vi "ATM.vi"() -> ()   [LabVIEW 2015]
uses:
  all data.ctl
  User data.ctl
  status.ctl
  user action.ctl
panel:
  out "error out":errorcluster
  in  "error in":errorcluster
  in  "Enter":bool
  in  "User Input":string
  in  "Right Buttons":T1
  out "Right Menu":T2
  in  "Left Buttons":T1
  out "Left Menu":T2
  in  "Card Simulator":bool
  out "ATM Messages":string
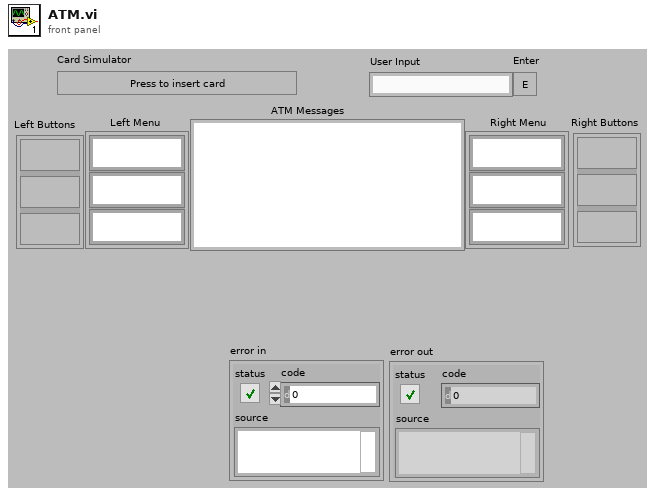
[diagram p1: front panel]
types:
  T1 = cluster{"Func Button":bool, "Func Button 2":bool, "Func Button 3":bool}
  T2 = cluster{"RFS String":string, "RFS String 2":string, "RFS String 3":string}
  T3 = enum8{"Enabled", "Disabled", "Disabled and Grayed Out"}
  T4 = typedef "all data.ctl" = cluster{"order":string, "Users":T5[], "user num":i32}
  T5 = typedef "User data.ctl" = cluster{"Code":string, "Name":string, "Surname":string, "Money":string}
  T6 = typedef "status.ctl" = enum16{"Get", "Set"}
  T7 = typedef "user action.ctl" = enum16{"Name", "Withdraw", "Deposit", "Balance"}
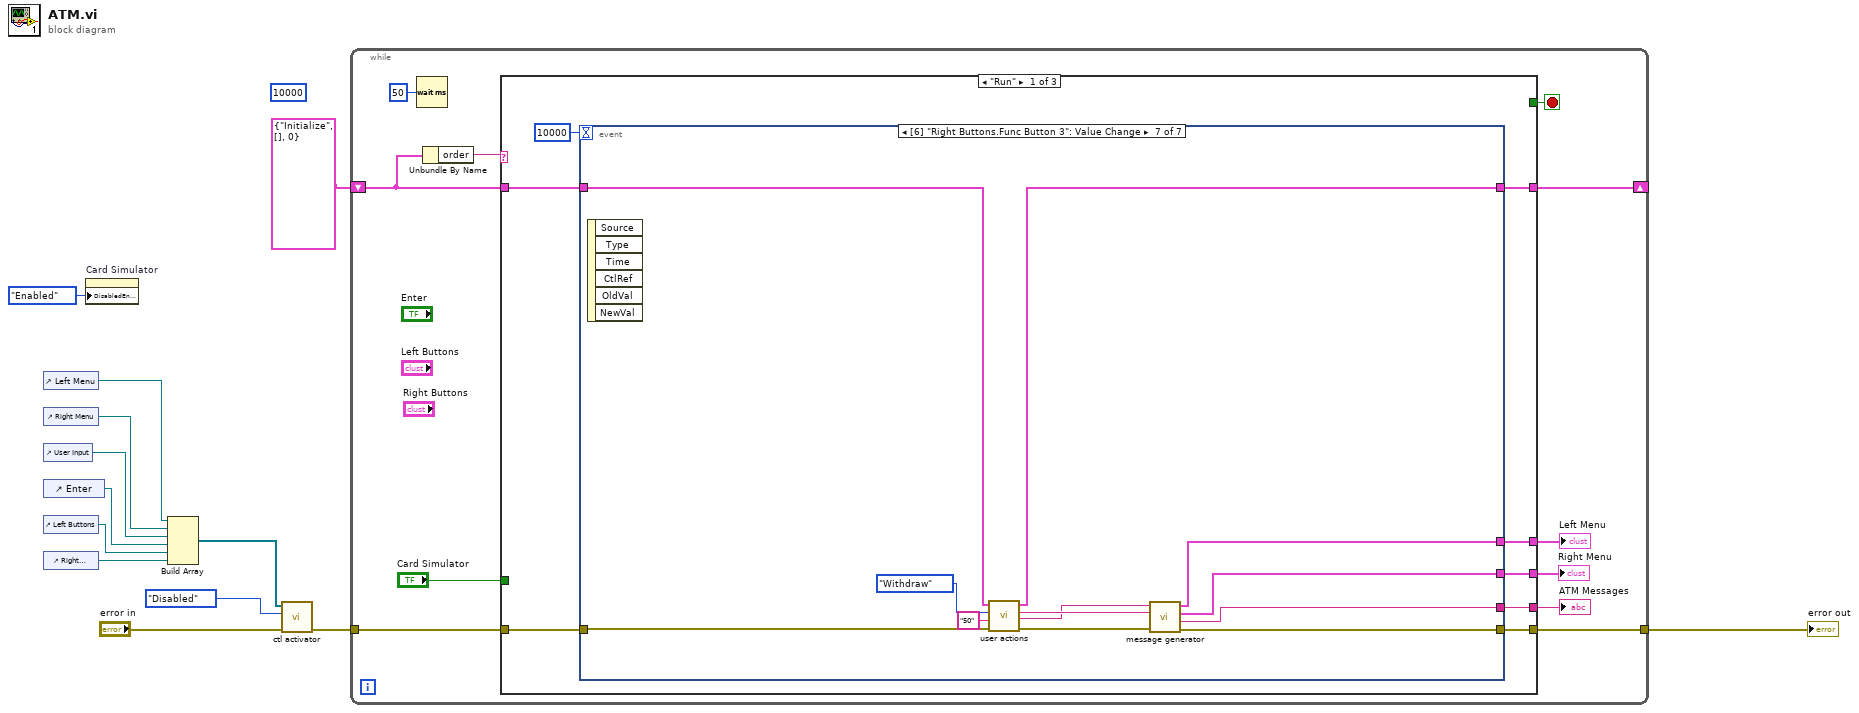
[diagram p0: block diagram]
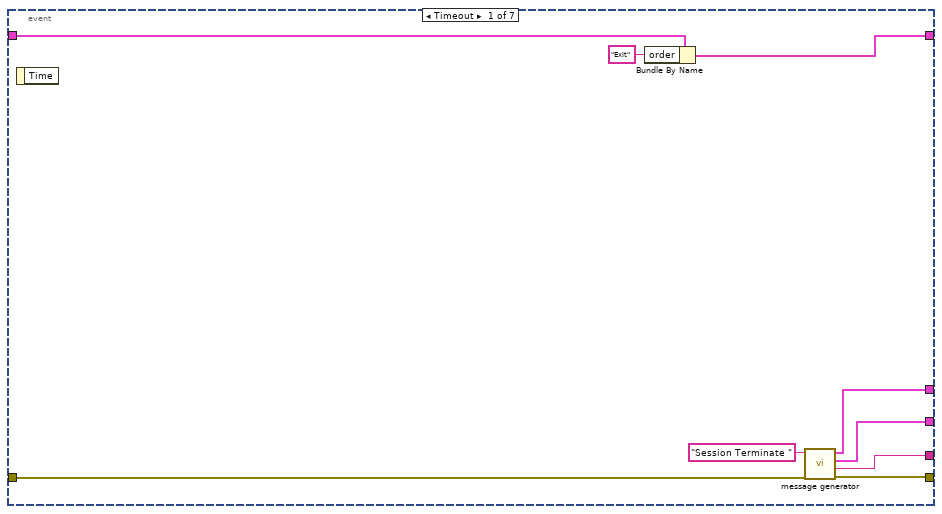
[diagram p2: hidden frame]
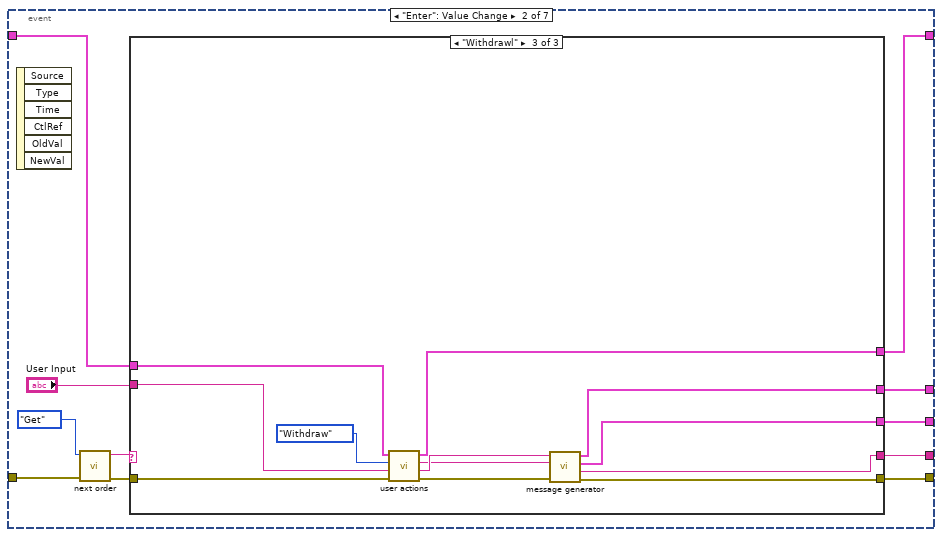
[diagram p3: hidden frame]
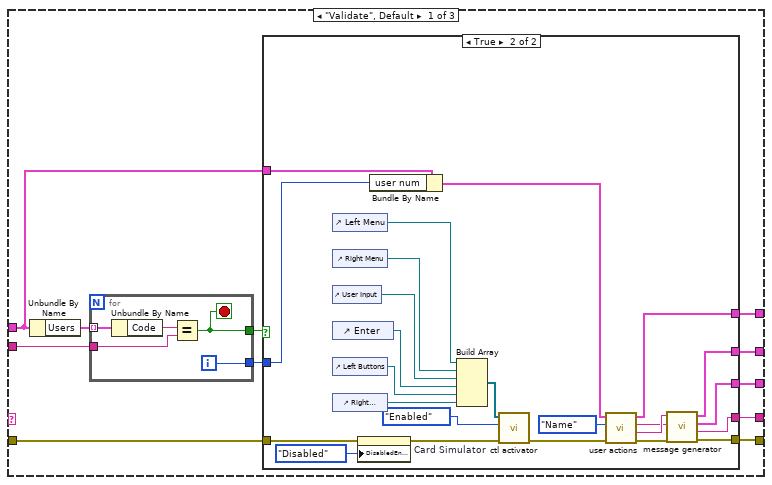
[diagram p4: hidden frame]
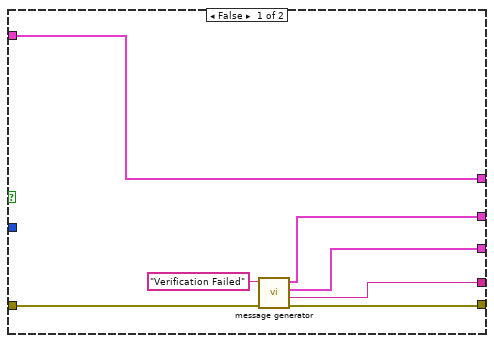
[diagram p5: hidden frame]
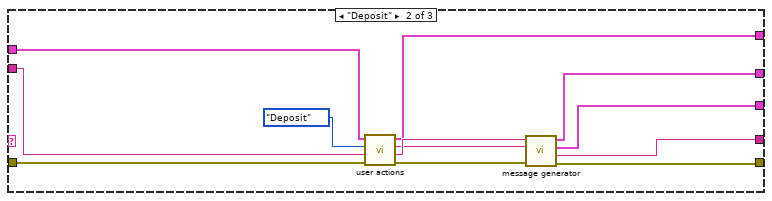
[diagram p6: hidden frame]
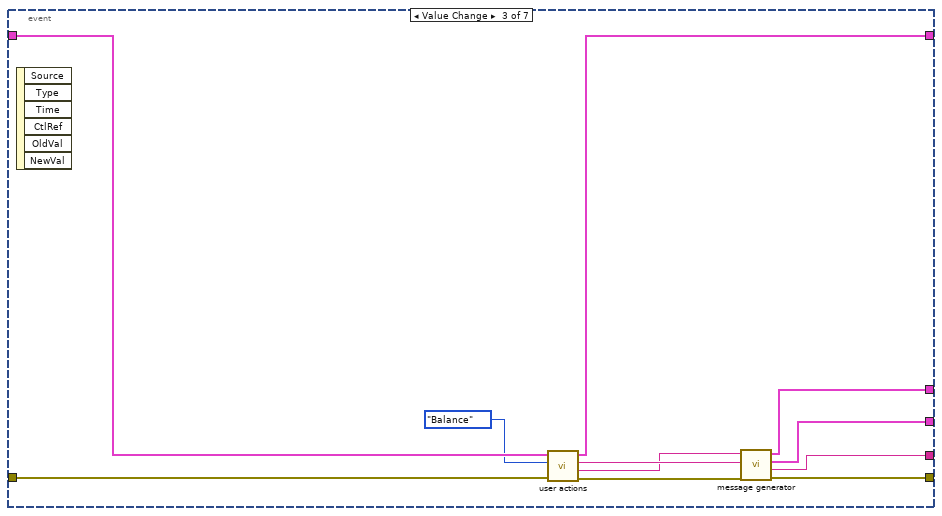
[diagram p7: hidden frame]
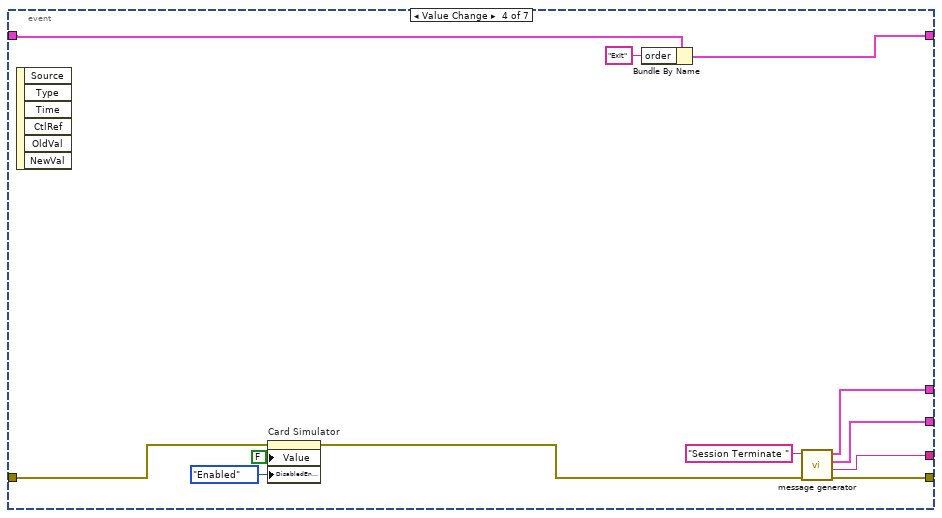
[diagram p8: hidden frame]
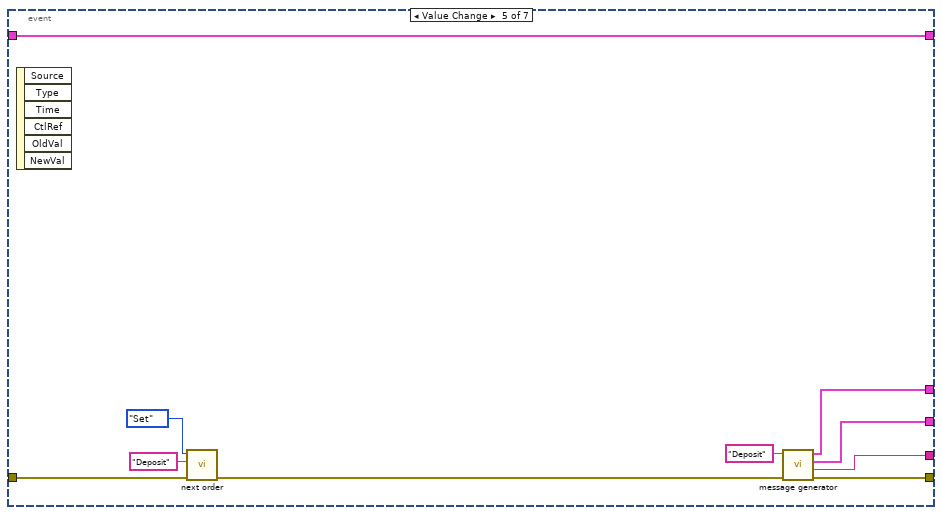
[diagram p9: hidden frame]
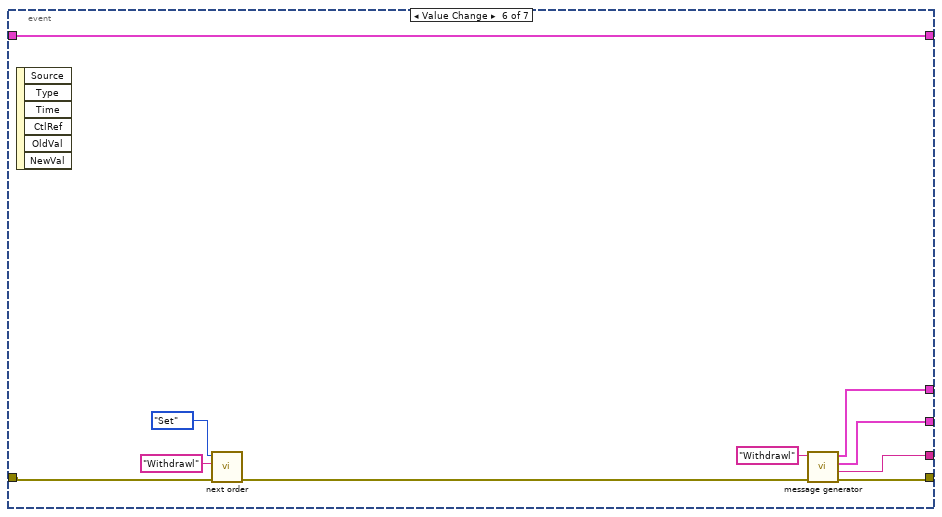
[diagram p10: hidden frame]
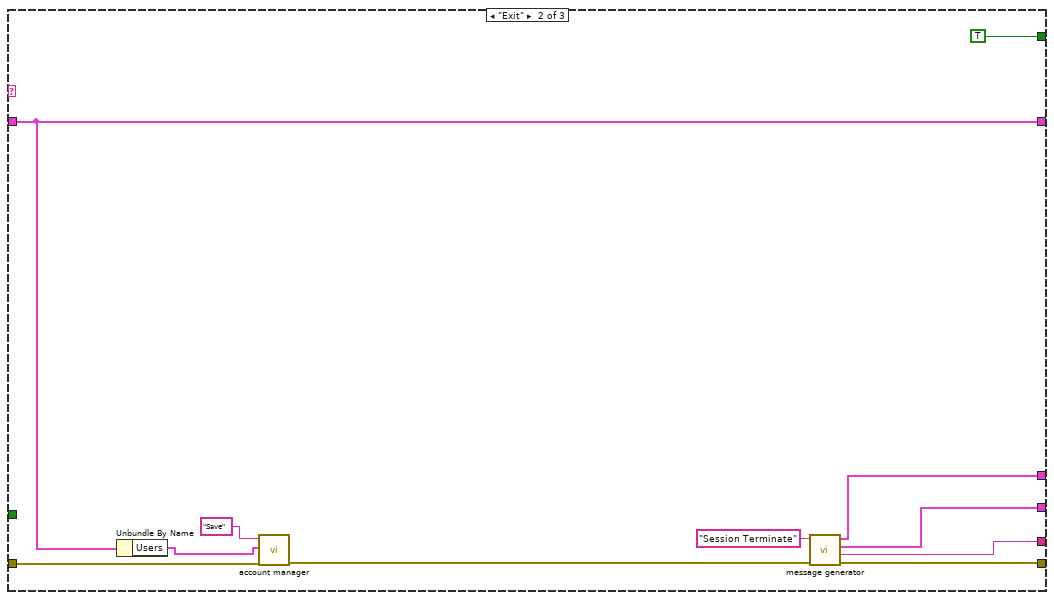
[diagram p11: hidden frame]
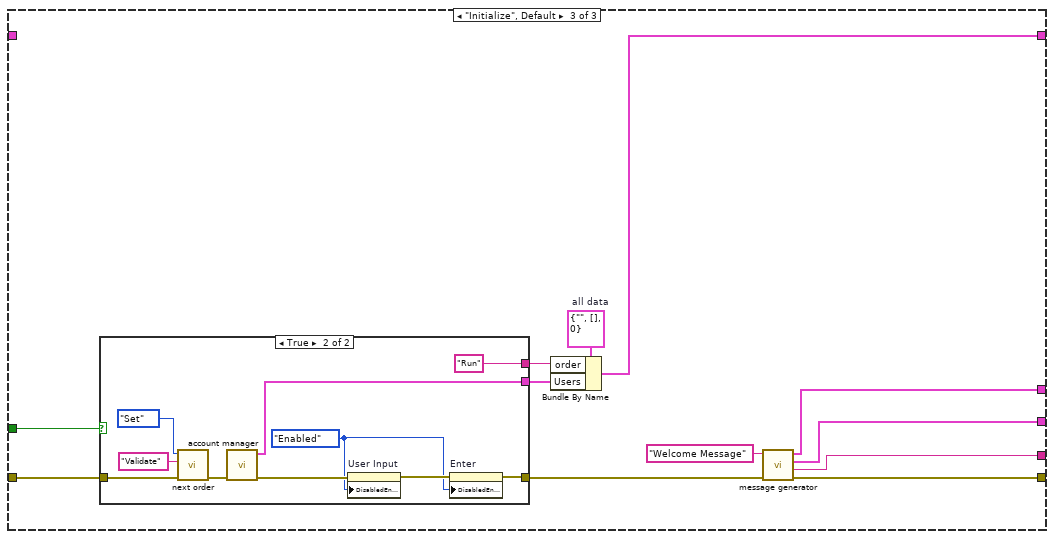
[diagram p12: hidden frame]
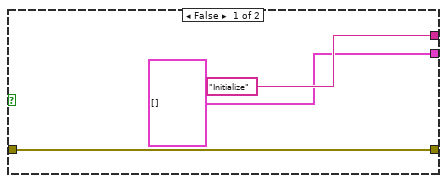
[diagram p13: hidden frame]
diagram:
  (unwired) 10000
  n1 = control-ref of="Left Menu"() -> (w4:refnum<vi>)
  n2 = control-ref of="Right Menu"() -> (w3:refnum<vi>)
  n3 = control-ref of="User Input"() -> (w5:refnum<vi>)
  n4 = control-ref of="Enter"() -> (w6:refnum<vi>)
  n5 = control-ref of="Left Buttons"() -> (w7:refnum<vi>)
  n6 = control-ref of="Right Buttons"() -> (w8:refnum<vi>)
  n7 = property on="Card Simulator" class="Bool (strict)"("DisabledEnum"=T3."Enabled" ("Disabled")) -> ()  [unwired: 2 in, 2 out]
  n8 = Build Array(w4, w3, w5, w6, w7, w8) -> (w2:refnum<vi>[])
  n9 = call "ctl activator.vi"("error in"="error in", "Disabled"=T3."Disabled", "Array"=w2) -> ("error out"=w10:errorcluster)  [unwired: 8 in]
  n10 = while {
    tunnel: w10 -> [w24]
    tunnel: [w21] -> w13
    shift-right: [w23] -> _
    shift-left: T4 {"order"="Initialize", "Users"=[], "user num"=0} ("all data") -> [w15]
    stop <- w16 stop-if-true
    n11 = Wait (ms)(milliseconds to wait=u32 50) -> ()  [unwired: 1 out]
    n12 = Unbundle By Name(w15) -> ("order"=w20:string)
    n13 = case shown="\"Run\"" w20 {
      tunnel: w24 -> [w32 w188 w200]
      tunnel: [w26 w186 w197] -> w23
      tunnel: "Card Simulator" -> [_ _ w196]
      tunnel: [w31 w183 w194] -> w21
      tunnel: [w28 w179 w192] -> w19
      tunnel: [w29 w180 w191] -> w18
      tunnel: [w30 w181 w190] -> w17
      tunnel: [_ TRUE _] -> w16
      tunnel: w15 -> [w27 w186 _]
      frame "Run" {
        n14 = event shown="[6] \"Right Buttons.Func Button 3\": Value Change" {
          selector: _ -> [_ _ _ _ _ _ _]
          dyn-events: _ -> [_ _ _ _ _ _ _]
          timeout: 10000 -> [_ _ _ _ _ _ _]
          tunnel: w32 -> [w41 w51 w133 w138 w154 w163 w173]
          tunnel: [w40 w46 w134 w144 w151 w162 w172] -> w31
          tunnel: [w38 w45 w124 w143 w148 w160 w169] -> w30
          tunnel: [w37 w44 w125 w142 w149 w159 w170] -> w29
          tunnel: [w36 w43 w126 w141 w150 w158 w171] -> w28
          tunnel: w27 -> [w35 w48 w131 w140 w147 w157 w168]
          tunnel: [w34 w47 w129 w139 w147 w157 w167] -> w26
          event Timeout {
            n15 = event-data() -> ()  [unwired: 1 in, 1 out]
            n16 = Bundle By Name(cluster=w35, "order"="Exit") -> (w34:T4)
            n17 = call "message generator.vi"("error in"=w41, "message"="Session Terminate ") -> ("error out"=w40:errorcluster, "Message"=w36:string, "Right Menu"=w37:T2, "Left Menu"=w38:T2)  [unwired: 6 in]
          }
          event "Enter": Value Change {
            n18 = event-data() -> ()  [unwired: 1 in, 6 out]
            n19 = call "next order.vi"("error in"=w51, "status"=status."Get") -> ("error out"=w50:errorcluster, "Order"=w49:string)  [unwired: 8 in]
            n20 = case shown="\"Withdrawl\"" w49 {
              tunnel: w50 -> [w62 w110 w121]
              tunnel: "User Input" -> [w63 w109 w114]
              tunnel: w48 -> [w59 w108 w115]
              tunnel: [w57 w103 w116] -> w47
              tunnel: [w53 w106 w120] -> w46
              tunnel: [w56 w102 w117] -> w45
              tunnel: [w55 w101 w118] -> w44
              tunnel: [w54 w100 w119] -> w43
              frame "Validate", Default {
                n21 = Unbundle By Name(w59) -> ("Users"=w60:T5[])
                n22 = for {
                  tunnel: w63 -> [w97]
                  tunnel: w60 -> [w99] mode=indexing
                  tunnel: [w95] -> w61
                  tunnel: [w96] -> w58
                  i -> [w96]
                  stop <- w95 stop-if-true
                  n23 = Unbundle By Name(w99) -> ("Code"=w98:string)
                  n24 = Equal?(x=w98, y=w97) -> (x = y?=w95:bool)
                }
                n25 = case shown="True" w61 {
                  tunnel: w62 -> [w69 w74]
                  tunnel: w59 -> [w70 w94]
                  tunnel: w58 -> [_ w93]
                  tunnel: [w70 w90] -> w57
                  tunnel: [w67 w85] -> w56
                  tunnel: [w66 w84] -> w55
                  tunnel: [w65 w83] -> w54
                  tunnel: [w64 w88] -> w53
                  frame False {
                    n26 = call "message generator.vi"("error in"=w69, "message"="Verification Failed") -> ("error out"=w64:errorcluster, "Message"=w65:string, "Right Menu"=w66:T2, "Left Menu"=w67:T2)  [unwired: 6 in]
                  }
                  frame True {
                    n27 = control-ref of="Left Menu"() -> (w77:refnum<vi>)
                    n28 = control-ref of="Right Menu"() -> (w76:refnum<vi>)
                    n29 = control-ref of="User Input"() -> (w78:refnum<vi>)
                    n30 = control-ref of="Enter"() -> (w79:refnum<vi>)
                    n31 = control-ref of="Left Buttons"() -> (w80:refnum<vi>)
                    n32 = control-ref of="Right Buttons"() -> (w81:refnum<vi>)
                    n33 = property on="Card Simulator" class="Bool (strict)"(error in=w74, "DisabledEnum"=T3."Disabled" ("Disabled")) -> (error out=w71:errorcluster)  [unwired: 1 in, 1 out]
                    n34 = Bundle By Name(cluster=w94, "user num"=w93) -> (w91:T4)
                    n35 = Build Array(w77, w76, w78, w79, w80, w81) -> (w75:refnum<vi>[])
                    n36 = call "ctl activator.vi"("error in"=w71, "Disabled"=T3."Enabled", "Array"=w75) -> ("error out"=w82:errorcluster)  [unwired: 8 in]
                    n37 = call "user actions.vi"("error in"=w82, "user action"=user_action."Name", "all data in"=w91) -> ("error out"=w89:errorcluster, "Message"=w87:string, "result"=w86:string, "all data out"=w90:T4)  [unwired: 5 in]
                    n38 = call "message generator.vi"("error in"=w89, "data"=w86, "message"=w87) -> ("error out"=w88:errorcluster, "Message"=w83:string, "Right Menu"=w84:T2, "Left Menu"=w85:T2)  [unwired: 5 in]
                  }
                }
              }
              frame "Deposit" {
                n39 = call "user actions.vi"("error in"=w110, "Amount"=w109, "user action"=user_action."Deposit", "all data in"=w108) -> ("error out"=w107:errorcluster, "Message"=w105:string, "result"=w104:string, "all data out"=w103:T4)  [unwired: 4 in]
                n40 = call "message generator.vi"("error in"=w107, "data"=w104, "message"=w105) -> ("error out"=w106:errorcluster, "Message"=w100:string, "Right Menu"=w101:T2, "Left Menu"=w102:T2)  [unwired: 5 in]
              }
              frame "Withdrawl" {
                n41 = call "user actions.vi"("error in"=w121, "Amount"=w114, "user action"=user_action."Withdraw", "all data in"=w115) -> ("error out"=w123:errorcluster, "Message"=w113:string, "result"=w112:string, "all data out"=w116:T4)  [unwired: 4 in]
                n42 = call "message generator.vi"("error in"=w123, "data"=w112, "message"=w113) -> ("error out"=w120:errorcluster, "Message"=w119:string, "Right Menu"=w118:T2, "Left Menu"=w117:T2)  [unwired: 5 in]
              }
            }
          }
          event "Left Buttons.Func Button 2": Value Change {
            n43 = event-data() -> ()  [unwired: 1 in, 6 out]
            n44 = call "user actions.vi"("error in"=w133, "user action"=user_action."Balance", "all data in"=w131) -> ("error out"=w132:errorcluster, "Message"=w127:string, "result"=w128:string, "all data out"=w129:T4)  [unwired: 5 in]
            n45 = call "message generator.vi"("error in"=w132, "data"=w128, "message"=w127) -> ("error out"=w134:errorcluster, "Message"=w126:string, "Right Menu"=w125:T2, "Left Menu"=w124:T2)  [unwired: 5 in]
          }
          event "Left Buttons.Func Button 3": Value Change {
            n46 = event-data() -> ()  [unwired: 1 in, 6 out]
            n47 = property on="Card Simulator" class="Bool (strict)"(error in=w138, "Value"=FALSE ("Card Simulator"), "DisabledEnum"=T3."Enabled" ("Disabled")) -> (error out=w137:errorcluster)  [unwired: 1 in, 1 out]
            n48 = Bundle By Name(cluster=w140, "order"="Exit") -> (w139:T4)
            n49 = call "message generator.vi"("error in"=w137, "message"="Session Terminate ") -> ("error out"=w144:errorcluster, "Message"=w141:string, "Right Menu"=w142:T2, "Left Menu"=w143:T2)  [unwired: 6 in]
          }
          event "Right Buttons.Func Button": Value Change {
            n50 = event-data() -> ()  [unwired: 1 in, 6 out]
            n51 = call "next order.vi"("error in"=w154, "Order"="Deposit", "status"=status."Set") -> ("error out"=w153:errorcluster)  [unwired: 7 in, 1 out]
            n52 = call "message generator.vi"("error in"=w153, "message"="Deposit") -> ("error out"=w151:errorcluster, "Message"=w150:string, "Right Menu"=w149:T2, "Left Menu"=w148:T2)  [unwired: 6 in]
          }
          event "Right Buttons.Func Button 2": Value Change {
            n53 = event-data() -> ()  [unwired: 1 in, 6 out]
            n54 = call "next order.vi"("error in"=w163, "Order"="Withdrawl", "status"=status."Set") -> ("error out"=w164:errorcluster)  [unwired: 7 in, 1 out]
            n55 = call "message generator.vi"("error in"=w164, "message"="Withdrawl") -> ("error out"=w162:errorcluster, "Message"=w158:string, "Right Menu"=w159:T2, "Left Menu"=w160:T2)  [unwired: 6 in]
          }
          event "Right Buttons.Func Button 3": Value Change {
            n56 = event-data() -> ()  [unwired: 1 in, 6 out]
            n57 = call "user actions.vi"("error in"=w173, "Amount"="50", "user action"=user_action."Withdraw", "all data in"=w168) -> ("error out"=w175:errorcluster, "Message"=w177:string, "result"=w178:string, "all data out"=w167:T4)  [unwired: 4 in]
            n58 = call "message generator.vi"("error in"=w175, "data"=w178, "message"=w177) -> ("error out"=w172:errorcluster, "Message"=w171:string, "Right Menu"=w170:T2, "Left Menu"=w169:T2)  [unwired: 5 in]
          }
        }
      }
      frame "Exit" {
        n59 = Unbundle By Name(w186) -> ("Users"=w185:T5[])
        n60 = call "account manager.vi"("error in"=w188, "Users"=w185, "action"="Save") -> ("error out"=w184:errorcluster)  [unwired: 7 in, 1 out]
        n61 = call "message generator.vi"("error in"=w184, "message"="Session Terminate") -> ("error out"=w183:errorcluster, "Message"=w179:string, "Right Menu"=w180:T2, "Left Menu"=w181:T2)  [unwired: 6 in]
      }
      frame "Initialize", Default {
        w201 = T4 {"order"="", "Users"=[], "user num"=0}  # all data
        n62 = case shown="True" w196 {
          tunnel: w200 -> [w204 w212]
          tunnel: [w204 w206] -> w195
          tunnel: [T5[] [] ("Users") w214] -> w199
          tunnel: ["Initialize" "Run"] -> w198
          frame False {
          }
          frame True {
            w205 = T3."Enabled" ("Disabled")
            n63 = call "next order.vi"("error in"=w212, "Order"="Validate", "status"=status."Set") -> ("error out"=w211:errorcluster)  [unwired: 7 in, 1 out]
            n64 = call "account manager.vi"("error in"=w211) -> ("error out"=w208:errorcluster, "Users"=w214:T5[])  [unwired: 9 in]
            n65 = property on="User Input" class="Str"(error in=w208, "DisabledEnum"=w205) -> (error out=w207:errorcluster)  [unwired: 1 in, 1 out]
            n66 = property on="Enter" class="Bool"(error in=w207, "DisabledEnum"=w205) -> (error out=w206:errorcluster)  [unwired: 1 in, 1 out]
          }
        }
        n67 = Bundle By Name(cluster=w201, "order"=w198, "Users"=w199) -> (w197:T4)
        n68 = call "message generator.vi"("error in"=w195, "message"="Welcome Message") -> ("error out"=w194:errorcluster, "Message"=w192:string, "Right Menu"=w191:T2, "Left Menu"=w190:T2)  [unwired: 6 in]
      }
    }
    "ATM Messages" <- w19
    "Left Menu" <- w17
    "Right Menu" <- w18
  }
  "error out" <- w13
